vi "Proiect Rn Toth David-Andrei 633 AB-Detectarea defectiunilor pieselor auto.vi"() -> ()   [LabVIEW 2024]
uses:
  <vilib>/vision/NI_Vision_Development_Module.lvlib
panel:
  in  "nr epoci":i32
  out "Status piesa":string
  in  "error in (no error) 2":errorcluster
  out "error out 2":errorcluster
  in  "Butonul de oprire":bool
  out "error out":errorcluster
  in  "error in (no error)":errorcluster
  in  "Calea imaginii care urmeaza sa fie verificata":path
  out "Imaginea finala":T1(plugin-control)
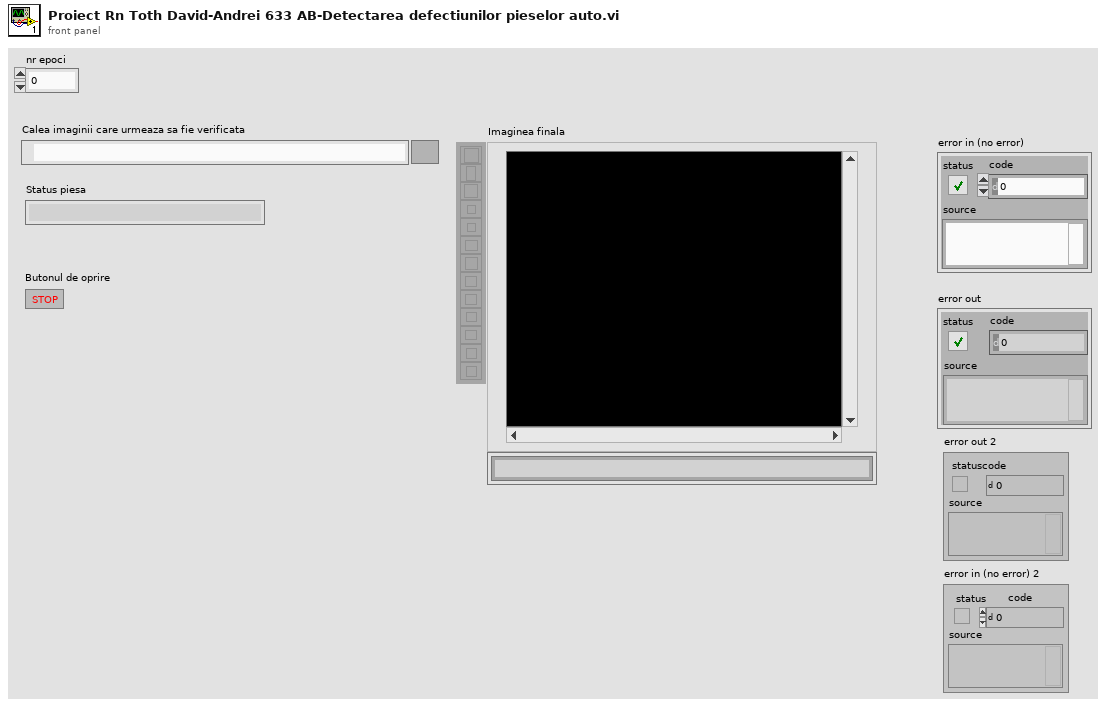
[diagram p1: front panel]
types:
  T1 = typedef "IMAQ Image.ctl" = refnum<image>
  T2 = enum32{"AutoM", "Close", "Dilate", "Erode", "Gradient", "Gradient out", "Gradient in", "Hit miss", "Open", "PClose", "POpen", "Thick", "Thin"}
  T3 = typedef "Image Type" = u32
  T4 = cluster{"Area":dbl, "Number of Holes":dbl, "Bounding Rect":cluster{"Left":dbl, "Top":dbl, "Right":dbl, "Bottom":dbl}, "Center of Mass":cluster{"X":dbl, "Y":dbl}, "Orientation":dbl, "Dimensions":cluster{"Width":dbl, "Height":dbl}}[]
  T5 = cluster{"Left":dbl, "Top":dbl, "Right":dbl, "Bottom":dbl}
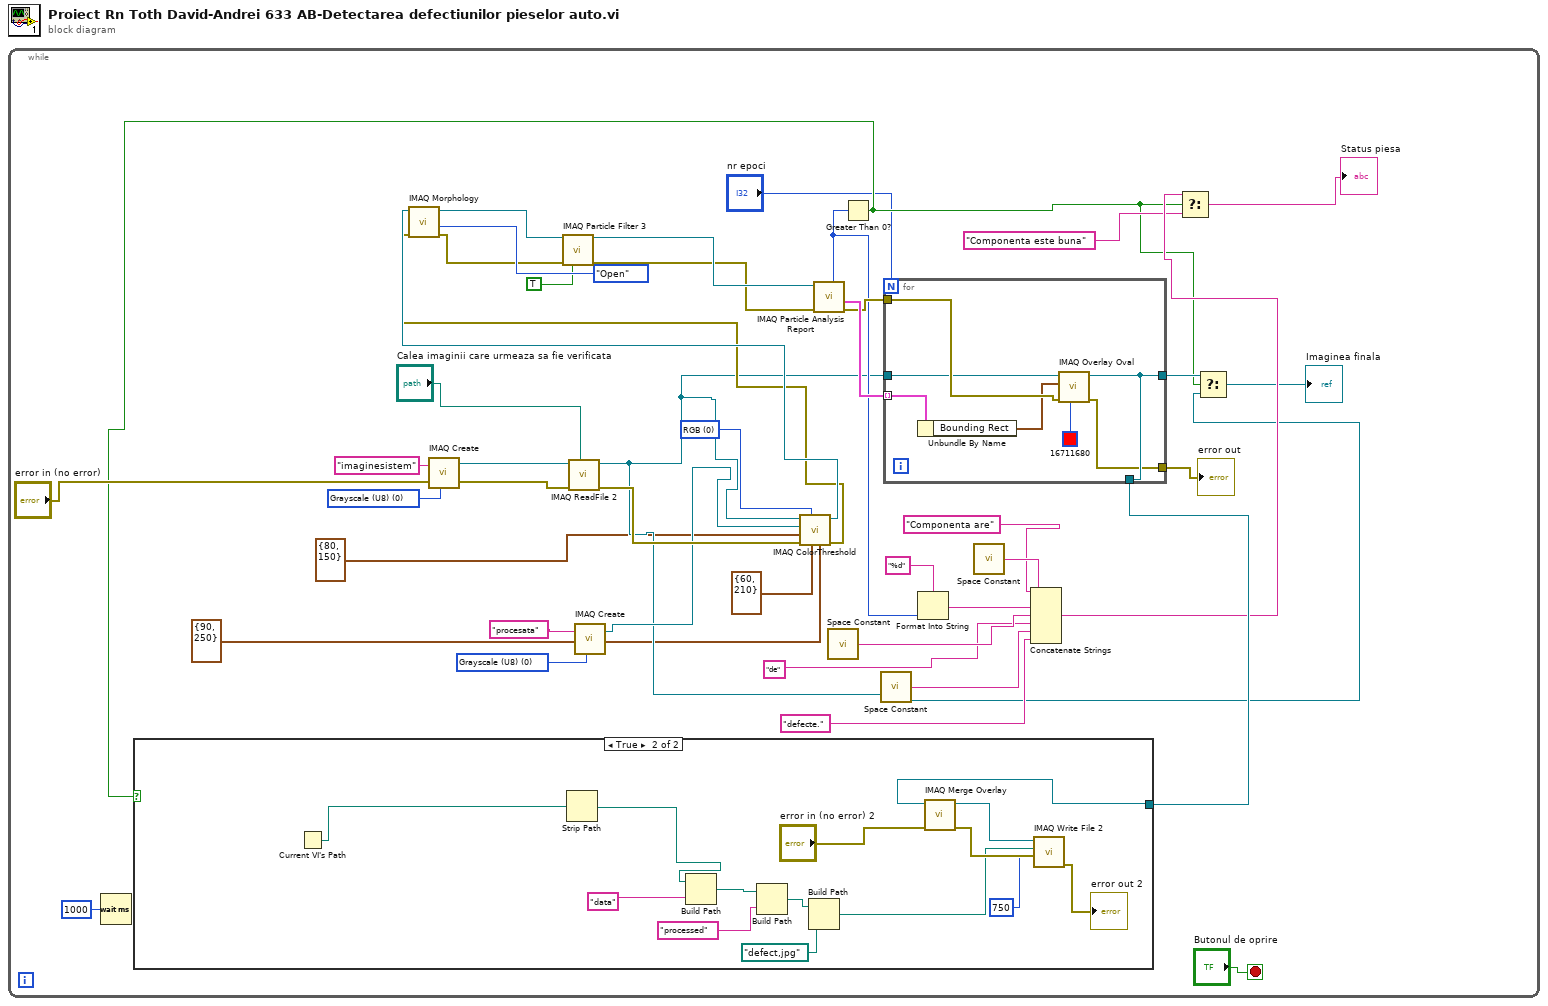
[diagram p0: block diagram]
diagram:
  n1 = while {
    stop <- "Butonul de oprire" stop-if-true
    w23 = u16 0 items=["RGB", "HSL", "HSV", "HSI"] ("Color Mode")
    w35 = T3 0 items=["Grayscale (U8)", "Grayscale (I16)", "Grayscale (SGL)", "Complex (CSG)", "RGB (U32)", "HSL (U32)", "RGB (U64)", "Grayscale (U16)"] ("Image Type")
    w44 = T3 0 items=["Grayscale (U8)", "Grayscale (I16)", "Grayscale (SGL)", "Complex (CSG)", "RGB (U32)", "HSL (U32)", "RGB (U64)", "Grayscale (U16)"] ("Image Type")
    n2 = Wait (ms)(milliseconds to wait=u32 1000) -> ()  [unwired: 1 out]
    n3 = call "IMAQ Create"("Image Name"="imaginesistem", "Image Type"=w44, "error in (no error)"="error in (no error)") -> ("New Image"=w42:T1, "error out"=w43:errorcluster)  [unwired: 2 in]
    n4 = call "IMAQ ReadFile 2"("File Path"="Calea imaginii care urmeaza sa fie verificata", "error in (no error)"=w43, "Image"=w42) -> ("error out"=w22:errorcluster, "Image Out"=w6:T1)  [unwired: 4 in, 3 out]
    n5 = call "IMAQ Create"("Image Name"="procesata", "Image Type"=w35) -> ("New Image"=w21:T1)  [unwired: 3 in, 1 out]
    n6 = call "IMAQ ColorThreshold"("Blue or Luma or Val or Inten Range"=cluster{"Lower value":i32, "Upper value":i32} {"Lower value"=90, "Upper value"=250}, "Green or Sat Range"=cluster{"Lower value":i32, "Upper value":i32} {"Lower value"=60, "Upper value"=210}, "Color Mode"=w23, "error in (no error)"=w22, "Red or Hue Range"=cluster{"Lower value":i32, "Upper value":i32} {"Lower value"=80, "Upper value"=150}, "Image Dst"=w21, "Image Src"=w6) -> ("error out"=w10:errorcluster, "Image Dst Out"=w12:T1)  [unwired: 3 in]
    n7 = call "IMAQ Morphology"("error in (no error)"=w10, "Operation"=T2."Open", "Image Src"=w12) -> ("error out"=w9:errorcluster, "Image Dst Out"=w14:T1)  [unwired: 7 in]
    n8 = call "IMAQ Particle Filter 3"("Image Src"=w14, "error in (no error)"=w9, "Reject Border? (F)"=TRUE) -> ("Image Dst Out"=w13:T1, "error out"=w11:errorcluster)  [unwired: 10 in, 1 out]
    n9 = call "IMAQ Particle Analysis Report"("error in (no error)"=w11, "Image"=w13) -> ("error out"=w38:errorcluster, "Particle Reports (Real-World)"=w40:T4, "Number of Particles"=w20:i32)  [unwired: 4 in, 3 out]
    n10 = call <vilib>:"Space Constant.vi"() -> ("String"=w28:string)
    n11 = Greater Than 0?(x=w20) -> (x > 0?=w5:bool)
    n12 = call <vilib>:"Space Constant.vi"() -> ("String"=w26:string)
    n13 = for {
      N: "nr epoci" -> [_]
      tunnel: w40 -> [w66] mode=indexing
      tunnel: [w62] -> w7
      tunnel: [w61] -> w39
      tunnel: w38 -> [w64]
      tunnel: w6 -> [w63]
      tunnel: [w62] -> w24
      n14 = Unbundle By Name(w66) -> ("Bounding Rect"=w60:T5)
      n15 = call "IMAQ Overlay Oval"("Color"=u32 16711680, "error in (no error)"=w64, "Bounding Rectangle"=w60, "Image"=w63) -> ("error out"=w61:errorcluster, "Image Out"=w62:T1)  [unwired: 6 in]
    }
    "error out" <- w39
    n16 = case shown="True" w5 {
      tunnel: w24 -> [_ w58]
      frame False {
      }
      frame True {
        n17 = Current VI's Path() -> (path=w53:path)
        n18 = Strip Path(path=w53) -> (stripped path=w52:path)  [unwired: 1 out]
        n19 = Build Path(base path=w52, name or relative path="data") -> (appended path=w50:path)
        n20 = Build Path(base path=w50, name or relative path="processed") -> (appended path=w48:path)
        n21 = Build Path(base path=w48, name or relative path=path "defect,jpg") -> (appended path=w47:path)
        n22 = call "IMAQ Merge Overlay"("error in (no error)"="error in (no error) 2", "Image Src"=w58) -> ("error out"=w59:errorcluster, "Image Dst Out"=w57:T1)  [unwired: 8 in]
        n23 = call-poly "IMAQ Write File 2"("error in (no error)"=w59, "Image Quality"=u32 750, "File Path"=w47, "Image"=w57) -> ("error out"=→"error out 2":errorcluster)  [unwired: 6 in, 1 out]
      }
    }
    n24 = Format Into String "Format Into String"(format string="%d", w20) -> (resulting string=w29:string)  [unwired: 2 in, 1 out]
    n25 = call <vilib>:"Space Constant.vi"() -> ("String"=w31:string)
    n26 = Concatenate Strings "Concatenate Strings"("Componenta are" ("string"), w31, w29, w28, "de", w26, "defecte." ("string")) -> (w18:string)
    n27 = Select(t=w18, s=w5, f="Componenta este buna") -> (s? t:f=→"Status piesa":string)
    n28 = Select(t=w7, s=w5, f=w6) -> (s? t:f=→"Imaginea finala":T1)
  }
